vi "Teleop.vi"(10 "Match Info":T1={"Autonomous Elapsed Seconds"=0.0, "TeleOp Elapsed Seconds"=0.0, "Disabled Elapsed Seconds"=0.0, "Visited Autonomous"=FALSE, "Visited TeleOp"=FALSE, "Visited Disabled"=FALSE, "Autonomous Settings"={"Autonomous Style"=enum."Independent", "VI Refnum"=refnum}}, 11 "Call Context":T2) -> ()   [LabVIEW 2020]
doc: "This VI is called for each TeleOp packet received from the DS where the robot is not disabled. It is often used to read from the joysticks and update I/O or to update setpoints for timed control loops. It should complete and return within 20 milliseconds or it may miss DS packets."
uses:
  <vilib>/Rock Robotics/WPI/DriverStation/WPI_DriverStationDerivedRobotMode.ctl
  <vilib>/Rock Robotics/WPI/DriverStation/WPI_DriverStationMatch Info.ctl
  <vilib>/Rock Robotics/WPI/Utilities/WPI_GetSetVariantRefNum.vi
  <vilib>/Rock Robotics/Network Tables/NT Read Boolean.vi
  <vilib>/Rock Robotics/Network Tables/NT Read Number.vi
  Variable BX.vi
  RX.vi
  LX.vi
panel:
  out "Sample Slider 0":dbl(slide) scale=0.0..5.0
  out "Sample Boolean 1":bool
  out "Sample Boolean 0":bool
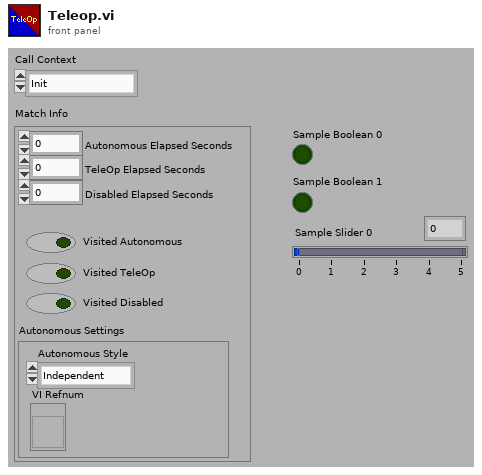
[diagram p1: front panel]
types:
  T1 = typedef "WPI_DriverStationMatch Info.ctl" = cluster{"Autonomous Elapsed Seconds":dbl, "TeleOp Elapsed Seconds":dbl, "Disabled Elapsed Seconds":dbl, "Visited Autonomous":bool, "Visited TeleOp":bool, "Visited Disabled":bool, "Autonomous Settings":cluster{"Autonomous Style":enum16{"Iterative", "Independent"}, "VI Refnum":refnum<vi>}}
  T2 = typedef "WPI_DriverStationDerivedRobotMode.ctl" = enum16{"Init", "Execute", "Stop"}
  T3 = typedef "WPI_JoystickDevRef.ctl" = cluster{"Device":T4}
  T4 = typedef "WPI_JoystickDeviceEnum.ctl" = enum16{"USB 0", "USB 1", "USB 2", "USB 3", "USB 4", "USB 5"}
  T5 = typedef "WPI_MotorControlDeviceRef.ctl" = cluster{"DeviceStatus":errorcluster, "Type":T6, "PWM":cluster{"PWM Channel":T7, "DeadBand":T8}, "CAN":cluster{"Device Number":u8, "SetOutput VI Ref":variant, "GetOutput VI Ref":variant, "Enable VI Ref":variant, "Disable VI Ref":variant, "Data":variant}, "Invert":bool, "DIO PWM":cluster{"PWM \"Enable\" Channel":T7, "DIOChannel":T9, "PWM Rate":dbl}}
  T6 = typedef "WPI_MotorControlType.ctl" = enum16{"PWM", "CAN", "DIO PWM"}
  T7 = typedef "FPGA_DIOPWMChannel.ctl" = enum8{"PWM 0", "PWM 1", "PWM 2", "PWM 3", "PWM 4", "PWM 5", "PWM 6", "PWM 7", "PWM 8", "PWM 9", "PWM MXP 0", "PWM MXP 1", "PWM MXP 2", "PWM MXP 3", "PWM MXP 4", "PWM MXP 5", "PWM MXP 6", "PWM MXP 7", "PWM MXP 8", "PWM MXP 9", "Invalid"}
  T8 = typedef "WPI_PWMDeadband.ctl" = cluster{"Name":string, "maxPositivePwm":i32, "minPositivePwm":i32, "centerPwm":i32, "maxNegativePwm":i32, "minNegativePwm":i32, "angularRange":u16}
  T9 = typedef "FPGA_DIOChannel.ctl" = enum8{"DIO 0", "DIO 1", "DIO 2", "DIO 3", "DIO 4", "DIO 5", "DIO 6", "DIO 7", "DIO 8", "DIO 9", "DIO MXP 0", "DIO MXP 1", "DIO MXP 2", "DIO MXP 3", "DIO MXP 4", "DIO MXP 5", "DIO MXP 6", "DIO MXP 7", "DIO MXP 8", "DIO MXP 9", "DIO MXP 10", "DIO MXP 11", "DIO MXP 12", "DIO MXP 13", "DIO MXP 14", "DIO MXP 15", "SPI Port CS1", "SPI Port CS2", "SPI Port CS3", "SPI Port MISO", "SPI Port MOSI", "Invalid"}
  T10 = typedef "WPI_RobotDriveDevRef.ctl" = cluster{"DevStatus":errorcluster, "Motors[]":T5[], "Square Inputs":bool, "Max Output":dbl}
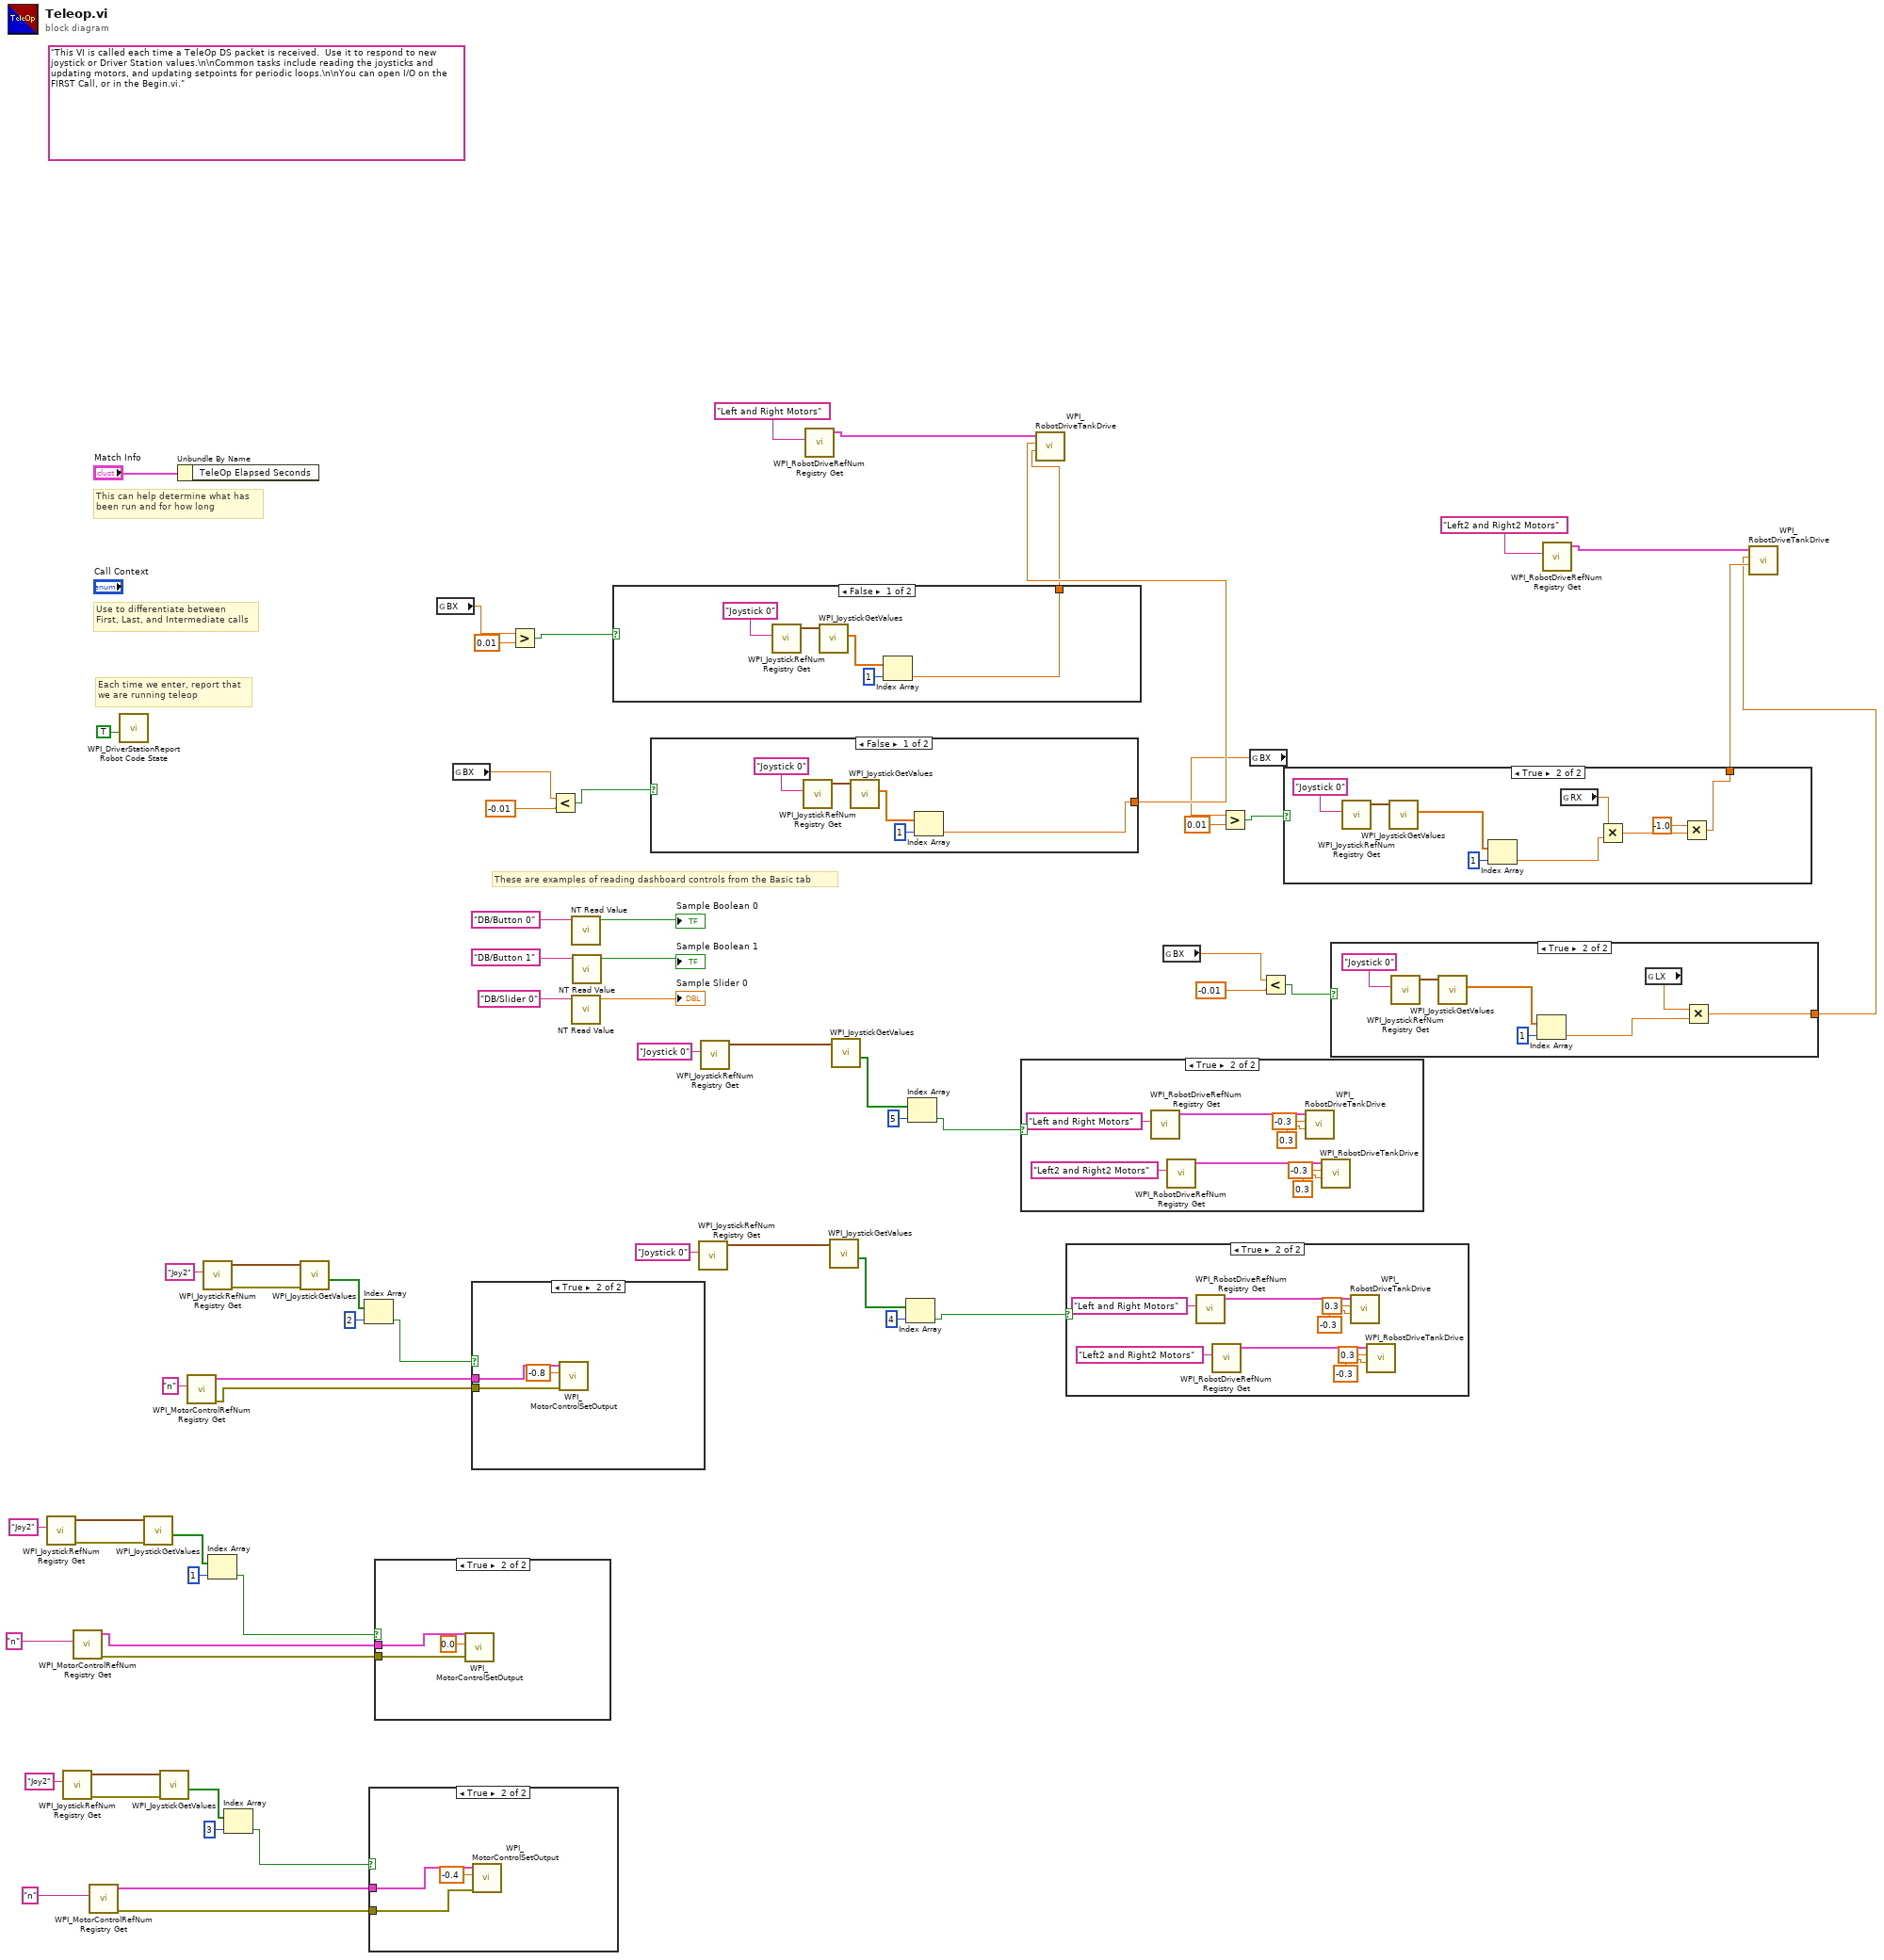
[diagram p0: block diagram]
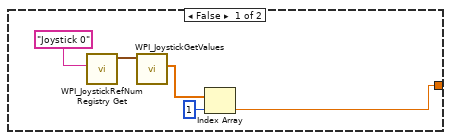
[diagram p7: hidden frame]
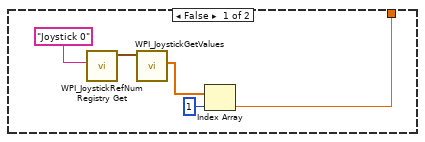
[diagram p8: hidden frame]
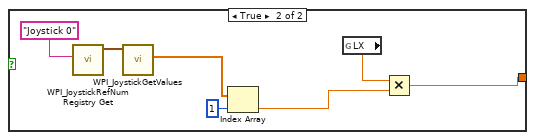
[diagram p9: hidden frame]
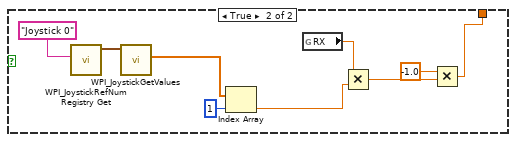
[diagram p10: hidden frame]
diagram:
  (unwired) "This VI is called each time a TeleOp DS packet is received.  Use it to respond to new joystick or Driver Station values.\n\nCommon tasks include reading the joysticks and updating motors, and updating setpoints for periodic loops.\n\nYou can open I/O on the FIRST Call, or in the Begin.vi."
  # "These are examples of reading dashboard controls from the Basic tab"
  # "Each time we enter, report that\nwe are running teleop"
  # "Use to differentiate between\nFirst, Last, and Intermediate calls"
  # "This can help determine what has\nbeen run and for how long"
  n1 = call <vilib>:"WPI_JoystickRefNum Registry Get.vi"("refnum name"="Joy2") -> ("error out"=w16:errorcluster, "JoystickDevRef"=w13:T3)  [unwired: 9 in]
  n2 = call <vilib>:"WPI_JoystickRefNum Registry Get.vi"("refnum name"="Joy2") -> ("error out"=w7:errorcluster, "JoystickDevRef"=w4:T3)  [unwired: 9 in]
  n3 = call <vilib>:"WPI_MotorControlRefNum Registry Get.vi"("refnum name"="n") -> ("error out"=w11:errorcluster, "MotorControlDevRef"=w10:T5)  [unwired: 9 in]
  n4 = call <vilib>:"WPI_MotorControlRefNum Registry Get.vi"("refnum name"="n") -> ("error out"=w1:errorcluster, "MotorControlDevRef"=w2:T5)  [unwired: 9 in]
  n5 = call <vilib>:"WPI_DriverStationReport Robot Code State.vi"("TeleOp"=TRUE ("Autonomous")) -> ()  [unwired: 10 in, 1 out]
  n6 = call <vilib>:"WPI_JoystickGetValues.vi"("error in (no error)"=w16, "JoystickDevRef"=w13) -> ("Buttons"=w14:bool[])  [unwired: 5 in, 4 out]
  n7 = call <vilib>:"WPI_JoystickGetValues.vi"("error in (no error)"=w7, "JoystickDevRef"=w4) -> ("Buttons"=w5:bool[])  [unwired: 5 in, 4 out]
  n8 = Unbundle By Name("Match Info") -> ()  [unwired: 1 out]
  n9 = call <vilib>:"WPI_MotorControlRefNum Registry Get.vi"("refnum name"="n") -> ("error out"=w20:errorcluster, "MotorControlDevRef"=w19:T5)  [unwired: 9 in]
  n10 = call <vilib>:"WPI_JoystickRefNum Registry Get.vi"("refnum name"="Joy2") -> ("error out"=w24:errorcluster, "JoystickDevRef"=w25:T3)  [unwired: 9 in]
  n11 = Index Array(array=w14, index=1) -> (element=w12:bool)
  n12 = Index Array(array=w5, index=3) -> (element=w3:bool)
  n13 = call <vilib>:"WPI_JoystickGetValues.vi"("error in (no error)"=w24, "JoystickDevRef"=w25) -> ("Buttons"=w22:bool[])  [unwired: 5 in, 4 out]
  n14 = Index Array(array=w22, index=2) -> (element=w21:bool)
  n15 = case shown="True" w3 {
    tunnel: w2 -> [_ w68]
    tunnel: w1 -> [_ w67]
    frame False {
    }
    frame True {
      n16 = call <vilib>:"WPI_MotorControlSetOutput.vi"("error in (no error)"=w67, "Output"=-0.4, "MotorControlDevRef"=w68) -> ()  [unwired: 6 in, 3 out]
    }
  }
  n17 = case shown="True" w12 {
    tunnel: w11 -> [_ w71]
    tunnel: w10 -> [_ w70]
    frame False {
    }
    frame True {
      n18 = call <vilib>:"WPI_MotorControlSetOutput.vi"("error in (no error)"=w71, "Output"=0.0, "MotorControlDevRef"=w70) -> ()  [unwired: 6 in, 3 out]
    }
  }
  n19 = global read "Variable BX.vi" "BX"() -> (w55:dbl)
  n20 = global read "Variable BX.vi" "BX"() -> (w52:dbl)
  n21 = case shown="True" w21 {
    tunnel: w20 -> [_ w74]
    tunnel: w19 -> [_ w73]
    frame False {
    }
    frame True {
      n22 = call <vilib>:"WPI_MotorControlSetOutput.vi"("error in (no error)"=w74, "Output"=-0.8, "MotorControlDevRef"=w73) -> ()  [unwired: 6 in, 3 out]
    }
  }
  n23 = Greater?(x=w55, y=0.01) -> (0:w53:bool)
  n24 = Less?(x=w52, y=-0.01) -> (x < y?=w50:bool)
  n25 = call-poly <vilib>:"NT Read Value.vi"("Name"="DB/Button 0" ("refnum name")) -> ("Boolean"=→"Sample Boolean 0":bool)  [unwired: 9 in, 1 out]
  n26 = call-poly <vilib>:"NT Read Value.vi"("Name"="DB/Slider 0" ("refnum name")) -> ("Numeric"=→"Sample Slider 0":dbl)  [unwired: 9 in, 1 out]
  n27 = call-poly <vilib>:"NT Read Value.vi"("Name"="DB/Button 1" ("refnum name")) -> ("Boolean"=→"Sample Boolean 1":bool)  [unwired: 9 in, 1 out]
  n28 = case shown="False" w53 {
    tunnel: [w75 w80] -> w46
    frame False {
      n29 = call <vilib>:"WPI_JoystickRefNum Registry Get.vi"("refnum name"="Joystick 0") -> ("JoystickDevRef"=w78:T3)  [unwired: 1 in, 9 out]
      n30 = call <vilib>:"WPI_JoystickGetValues.vi"("JoystickDevRef"=w78) -> ("Axes"=w79:dbl[])  [unwired: 6 in, 4 out]
      n31 = Index Array(array=w79, index=1) -> (element=w75:dbl)
    }
    frame True {
      n32 = call <vilib>:"WPI_JoystickRefNum Registry Get.vi"("refnum name"="Joystick 0") -> ("JoystickDevRef"=w86:T3)  [unwired: 1 in, 9 out]
      n33 = call <vilib>:"WPI_JoystickGetValues.vi"("JoystickDevRef"=w86) -> ("Axes"=w84:dbl[])  [unwired: 6 in, 4 out]
      n34 = Index Array(array=w84, index=1) -> (element=w83:dbl)
      n35 = global read "RX.vi" "RX"() -> (w87:dbl)
      n36 = Multiply(x=w87, y=w83) -> (x*y=w82:dbl)
      n37 = Multiply(x=-1.0, y=w82) -> (x*y=w80:dbl)
    }
  }
  n38 = case shown="False" w50 {
    tunnel: [w89 w94] -> w47
    frame False {
      n39 = call <vilib>:"WPI_JoystickRefNum Registry Get.vi"("refnum name"="Joystick 0") -> ("JoystickDevRef"=w92:T3)  [unwired: 1 in, 9 out]
      n40 = call <vilib>:"WPI_JoystickGetValues.vi"("JoystickDevRef"=w92) -> ("Axes"=w93:dbl[])  [unwired: 6 in, 4 out]
      n41 = Index Array(array=w93, index=1) -> (element=w89:dbl)
    }
    frame True {
      n42 = call <vilib>:"WPI_JoystickRefNum Registry Get.vi"("refnum name"="Joystick 0") -> ("JoystickDevRef"=w99:T3)  [unwired: 1 in, 9 out]
      n43 = call <vilib>:"WPI_JoystickGetValues.vi"("JoystickDevRef"=w99) -> ("Axes"=w97:dbl[])  [unwired: 6 in, 4 out]
      n44 = Index Array(array=w97, index=1) -> (element=w95:dbl)
      n45 = global read "LX.vi" "LX"() -> (w96:dbl)
      n46 = Multiply(x=w96, y=w95) -> (x*y=w94:dbl)
    }
  }
  n47 = call <vilib>:"WPI_JoystickRefNum Registry Get.vi"("refnum name"="Joystick 0") -> ("JoystickDevRef"=w36:T3)  [unwired: 9 in, 1 out]
  n48 = call <vilib>:"WPI_JoystickRefNum Registry Get.vi"("refnum name"="Joystick 0") -> ("JoystickDevRef"=w32:T3)  [unwired: 9 in, 1 out]
  n49 = call <vilib>:"WPI_RobotDriveRefNum Registry Get.vi"("refnum name"="Left and Right Motors") -> ("RobotDriveDevRef"=w56:T10)  [unwired: 1 in, 9 out]
  n50 = call <vilib>:"WPI_JoystickGetValues.vi"("JoystickDevRef"=w36) -> ("Buttons"=w35:bool[])  [unwired: 6 in, 4 out]
  n51 = call <vilib>:"WPI_JoystickGetValues.vi"("JoystickDevRef"=w32) -> ("Buttons"=w31:bool[])  [unwired: 6 in, 4 out]
  n52 = Index Array(array=w35, index=4) -> (element=w28:bool)
  n53 = Index Array(array=w31, index=5) -> (element=w29:bool)
  n54 = case shown="True" w29 {
    frame False {
    }
    frame True {
      n55 = call <vilib>:"WPI_RobotDriveRefNum Registry Get.vi"("refnum name"="Left and Right Motors") -> ("RobotDriveDevRef"=w108:T10)  [unwired: 9 in, 1 out]
      n56 = call <vilib>:"WPI_RobotDriveRefNum Registry Get.vi"("refnum name"="Left2 and Right2 Motors") -> ("RobotDriveDevRef"=w107:T10)  [unwired: 9 in, 1 out]
      n57 = call <vilib>:"WPI_RobotDriveTankDrive.vi"("Right axis value"=0.3, "Left axis value"=-0.3, "RobotDriveDevRef"=w108) -> ()  [unwired: 6 in, 3 out]
      n58 = call <vilib>:"WPI_RobotDriveTankDrive.vi"("Right axis value"=0.3, "Left axis value"=-0.3, "RobotDriveDevRef"=w107) -> ()  [unwired: 6 in, 3 out]
    }
  }
  n59 = call <vilib>:"WPI_RobotDriveTankDrive.vi"("Right axis value"=w46, "Left axis value"=w47, "RobotDriveDevRef"=w56) -> ()  [unwired: 6 in, 3 out]
  n60 = case shown="True" w28 {
    frame False {
    }
    frame True {
      n61 = call <vilib>:"WPI_RobotDriveRefNum Registry Get.vi"("refnum name"="Left and Right Motors") -> ("RobotDriveDevRef"=w116:T10)  [unwired: 9 in, 1 out]
      n62 = call <vilib>:"WPI_RobotDriveRefNum Registry Get.vi"("refnum name"="Left2 and Right2 Motors") -> ("RobotDriveDevRef"=w115:T10)  [unwired: 9 in, 1 out]
      n63 = call <vilib>:"WPI_RobotDriveTankDrive.vi"("Right axis value"=-0.3, "Left axis value"=0.3, "RobotDriveDevRef"=w116) -> ()  [unwired: 6 in, 3 out]
      n64 = call <vilib>:"WPI_RobotDriveTankDrive.vi"("Right axis value"=-0.3, "Left axis value"=0.3, "RobotDriveDevRef"=w115) -> ()  [unwired: 6 in, 3 out]
    }
  }
  n65 = global read "Variable BX.vi" "BX"() -> (w42:dbl)
  n66 = global read "Variable BX.vi" "BX"() -> (w45:dbl)
  n67 = Greater?(x=w45, y=0.01) -> (0:w43:bool)
  n68 = Less?(x=w42, y=-0.01) -> (x < y?=w40:bool)
  n69 = case shown="True" w43 {
    tunnel: [w117 w122] -> w39
    frame False {
      n70 = call <vilib>:"WPI_JoystickRefNum Registry Get.vi"("refnum name"="Joystick 0") -> ("JoystickDevRef"=w120:T3)  [unwired: 1 in, 9 out]
      n71 = call <vilib>:"WPI_JoystickGetValues.vi"("JoystickDevRef"=w120) -> ("Axes"=w121:dbl[])  [unwired: 6 in, 4 out]
      n72 = Index Array(array=w121, index=1) -> (element=w117:dbl)
    }
    frame True {
      n73 = call <vilib>:"WPI_JoystickRefNum Registry Get.vi"("refnum name"="Joystick 0") -> ("JoystickDevRef"=w128:T3)  [unwired: 1 in, 9 out]
      n74 = call <vilib>:"WPI_JoystickGetValues.vi"("JoystickDevRef"=w128) -> ("Axes"=w126:dbl[])  [unwired: 6 in, 4 out]
      n75 = Index Array(array=w126, index=1) -> (element=w125:dbl)
      n76 = global read "RX.vi" "RX"() -> (w129:dbl)
      n77 = Multiply(x=w129, y=w125) -> (x*y=w124:dbl)
      n78 = Multiply(x=-1.0, y=w124) -> (x*y=w122:dbl)
    }
  }
  n79 = case shown="True" w40 {
    tunnel: [w131 w136] -> w38
    frame False {
      n80 = call <vilib>:"WPI_JoystickRefNum Registry Get.vi"("refnum name"="Joystick 0") -> ("JoystickDevRef"=w134:T3)  [unwired: 1 in, 9 out]
      n81 = call <vilib>:"WPI_JoystickGetValues.vi"("JoystickDevRef"=w134) -> ("Axes"=w135:dbl[])  [unwired: 6 in, 4 out]
      n82 = Index Array(array=w135, index=1) -> (element=w131:dbl)
    }
    frame True {
      n83 = call <vilib>:"WPI_JoystickRefNum Registry Get.vi"("refnum name"="Joystick 0") -> ("JoystickDevRef"=w141:T3)  [unwired: 1 in, 9 out]
      n84 = call <vilib>:"WPI_JoystickGetValues.vi"("JoystickDevRef"=w141) -> ("Axes"=w139:dbl[])  [unwired: 6 in, 4 out]
      n85 = Index Array(array=w139, index=1) -> (element=w137:dbl)
      n86 = global read "LX.vi" "LX"() -> (w138:dbl)
      n87 = Multiply(x=w138, y=w137) -> (x*y=w136:dbl)
    }
  }
  n88 = call <vilib>:"WPI_RobotDriveRefNum Registry Get.vi"("refnum name"="Left2 and Right2 Motors") -> ("RobotDriveDevRef"=w48:T10)  [unwired: 1 in, 9 out]
  n89 = call <vilib>:"WPI_RobotDriveTankDrive.vi"("Right axis value"=w39, "Left axis value"=w38, "RobotDriveDevRef"=w48) -> ()  [unwired: 6 in, 3 out]
